vi "Convert I2C Data & Buffer.vi"(8 "error in (no error)":errorcluster, 11 "Data":u8[](array[numeric])) -> (0 "error out":errorcluster)   [LabVIEW 2025, in "I2C Bus Monitor UI.lvlib"]
uses:
  I2C Bus Monitor UI.lvlib
  Table Buffer - Enqueue.vi
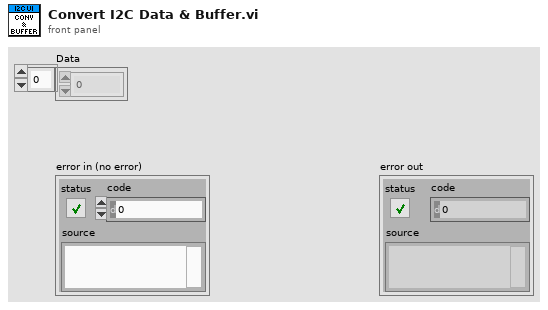
[diagram p1: front panel]
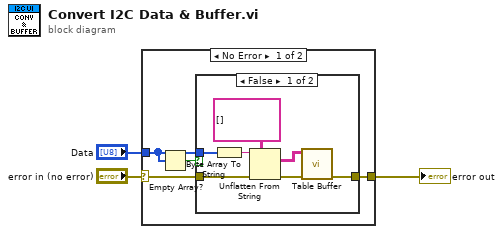
[diagram p0: block diagram]
diagram:
  n1 = case shown="No Error" "error in (no error)" {
    selector: "error in (no error)" -> [w4 w16]
    tunnel: [w7 w16] -> w3
    tunnel: "Data" -> [w6 _]
    frame No Error {
      n2 = Empty Array?(array=w6) -> (empty?=w5:bool)
      n3 = case shown="False" w5 {
        tunnel: w4 -> [w9 w15]
        tunnel: w6 -> [w12 _]
        tunnel: [w10 w15] -> w7
        frame False {
          n4 = Byte Array To String(unsigned byte array=w12) -> (string=w13:string)
          n5 = Unflatten From String(type=string[][] [] ("Fetched I2C Messages"), binary string=w13, error in (no error)=w9) -> (value=w8:string[][], error out=w11:errorcluster)  [unwired: 2 in, 1 out]
          n6 = call-poly "Table Buffer.vi"("error in (no error)"=w11, "Data"=w8) -> ("error out"=w10:errorcluster)  [unwired: 9 in]
        }
        frame True {
        }
      }
    }
    frame Error {
    }
  }
  "error out" <- w3
